vi "Event Self Alias.vi"(11 "Hello World Queue in":refnum<class "Hello World Queue.lvclass">) -> (2 "Event Self Alias":string)   [LabVIEW 2021, in "Hello World Queue.lvlib" / "Hello World Queue.lvclass"]
uses:
  Hello World Queue.lvclass
  Hello World Queue.lvclass/Hello World Queue.ctl
  jettl/jettl/Queue Actor/Queue Actor.lvclass
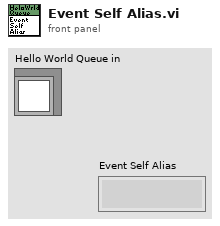
[diagram p1: front panel]
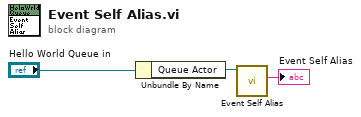
[diagram p0: block diagram]
diagram:
  n1 = Unbundle By Name("Hello World Queue in") -> ("Queue Actor"=w2:refnum<class "Queue Actor.lvclass">)
  n2 = call-dynamic "Event Self Alias.vi"("Actor in"=w2) -> ("Event Self Alias"=→"Event Self Alias":string)  [unwired: 10 in]
